vi "System_Guide-plot.vi"(6 "Time In":i32, 8 "Temperature Sync":i32, 9 "Temp Band % (e.g. 1%=1.01)":dbl=1.04, 10 "Mean(Off)/Interval(On)":bool, 11 "TempGuide":bool) -> (0 "Graph 4":dbl, 1 "Graph 3":dbl, 2 "Graph 2":dbl, 3 "Graph 1":dbl, 4 "Time out":i32)   [LabVIEW 2014]
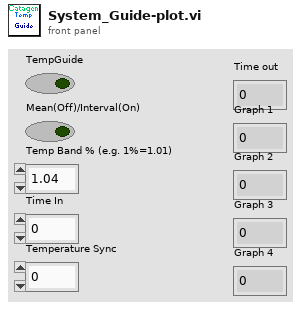
[diagram p1: front panel]
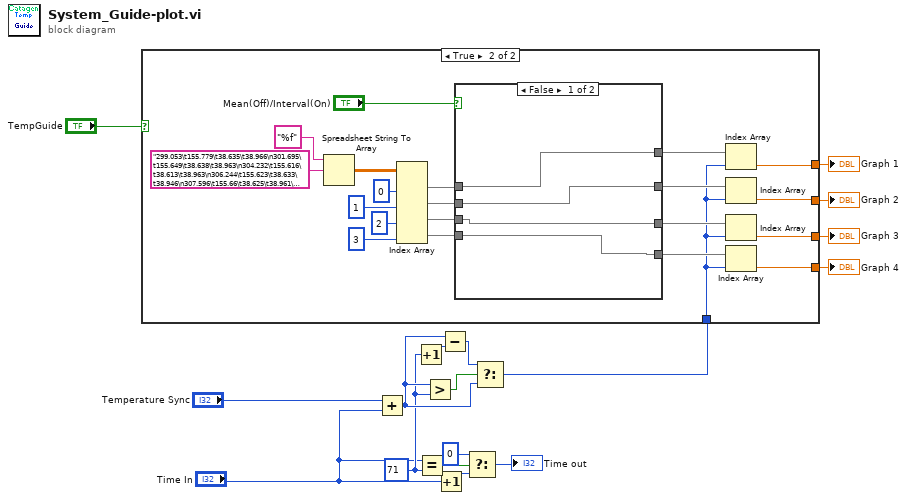
[diagram p0: block diagram]
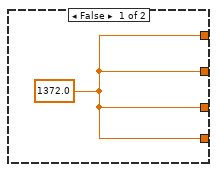
[diagram p2: hidden frame]
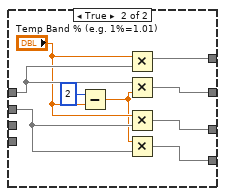
[diagram p3: hidden frame]
diagram:
  w8 = 71 ("y")
  n1 = Add(x="Temperature Sync", y="Time In") -> (x+y=w10:i32)
  n2 = Increment(x=w8) -> (x+1=w9:i32)
  n3 = Equal?(x="Time In", y=w8) -> (x = y?=w15:bool)
  n4 = Greater?(x=w10, y=w8) -> (0:w12:bool)
  n5 = Increment(x="Time In") -> (x+1=w13:i32)
  n6 = Subtract(x=w10, y=w9) -> (x-y=w11:i32)
  n7 = Select(t=0, s=w15, f=w13) -> (s? t:f=→"Time out":i32)
  n8 = Select(t=w11, s=w12, f=w10) -> (s? t:f=w7:i32)
  n9 = case shown="True" "TempGuide" {
    tunnel: w7 -> [_ w28]
    tunnel: [w18 w24] -> w4
    tunnel: [w18 w25] -> w3
    tunnel: [w18 w27] -> w2
    tunnel: [w18 w26] -> w1
    frame False {
      w18 = 1372.0
    }
    frame True {
      n10 = Spreadsheet String To Array(format string="%f", spreadsheet string="299.053\t155.779\t38.635\t38.966\n301.695\t155.649\t38.638\t38.963\n304.232\t155.616\t38.613\t38.963\n306.244\t155.623\t38.633\t38.946\n307.596\t155.66\t38.625\t38.961\n308.294\t155.857\t38.658\t38.928\n309.648\t155.893\t38.653\t38.934\n310.139\t156.057\t38.631\t38.949\n310.91\t156.073\t38.635\t38.976\n311.337\t156.182\t38.656\t38.934\n311.557\t156.297\t38.638\t38.927\n311.735\t156.496\t38.648\t38.94\n311.331\t156.331\t38.645\t38.933\n312.349\t156.573\t38.634\t38.926\n311.548\t156.657\t38.596\t38.866\n312.25\t156.94\t38.626\t38.938\n311.486\t157.037\t38.596\t38.93\n312.27\t157.108\t38.598\t38.918\n312.09\t157.285\t38.606\t38.939\n312.391\t157.179\t38.581\t38.912\n312.189\t157.496\t38.586\t38.923\n312.296\t157.418\t38.631\t38.956\n312.639\t157.483\t38.634\t38.91\n312.707\t157.778\t38.617\t38.926\n312.797\t157.869\t38.605\t38.919\n312.125\t157.953\t38.624\t38.884\n313.128\t158.062\t38.639\t38.911\n312.284\t158.157\t38.638\t38.893\n309.138\t158.378\t38.647\t38.906\n306.75\t158.387\t38.63\t38.911\n304.544\t158.237\t38.642\t38.928\n302.831\t158.006\t38.611\t38.891\n299.558\t157.813\t38.645\t38.947\n295.464\t157.413\t38.641\t38.929\n292.116\t157.055\t38.62\t38.906\n295.531\t156.58\t38.628\t38.923\n299.517\t156.284\t38.607\t38.929\n302.577\t156.271\t38.601\t38.931\n304.642\t156.227\t38.626\t38.915\n306.593\t156.238\t38.633\t38.915\n307.747\t156.343\t38.65\t38.916\n309.226\t156.368\t38.641\t38.948\n309.948\t156.588\t38.635\t38.919\n310.419\t156.708\t38.634\t38.967\n311.032\t156.802\t38.648\t39.004\n311.277\t156.957\t38.642\t38.968\n311.732\t156.994\t38.652\t38.916\n311.925\t157.11\t38.632\t38.973\n312.166\t157.279\t38.622\t38.956\n312.254\t157.296\t38.632\t38.966\n312.16\t157.492\t38.627\t38.961\n312.506\t157.536\t38.651\t38.976\n311.985\t157.508\t38.678\t38.968\n312.57\t157.727\t38.645\t38.98\n311.954\t157.632\t38.616\t38.957\n312.228\t157.895\t38.662\t38.966\n312.292\t157.836\t38.639\t38.965\n312.511\t157.872\t38.64\t38.993\n312.269\t157.969\t38.658\t38.981\n312.346\t158.137\t38.626\t38.935\n312.643\t158.208\t38.656\t38.966\n312.486\t158.2\t38.651\t38.971\n312.174\t158.203\t38.627\t38.906\n310.471\t158.505\t38.611\t38.983\n307.38\t158.432\t38.596\t38.972\n305.591\t158.343\t38.599\t38.974\n302.907\t158.133\t38.597\t38.927\n300.261\t157.782\t38.638\t38.94\n296.384\t157.418\t38.615\t38.979\n292.863\t156.943\t38.643\t38.943\n289.549\t156.606\t38.622\t39.006\n293.546\t156.064\t38.646\t39.006") -> (array=w38:dbl[][])  [unwired: 2 in]
      n11 = Index Array(array=w38, index (col) #1=0 ("disabled index (col)"), index (col) #2=1 ("disabled index (col)"), index (col) #3=2 ("index (col)"), index (col) #4=3 ("index (col)")) -> (element #1=w35:dbl[], element #2=w34:dbl[], element #3=w22:dbl[], element #4=w21:dbl[])  [unwired: 4 in]
      n12 = case shown="False" "Mean(Off)/Interval(On)" {
        tunnel: w35 -> [w43 w49]
        tunnel: w34 -> [w42 w46]
        tunnel: [w41 w44] -> w33
        tunnel: [w40 w48] -> w32
        tunnel: [w42 w50] -> w30
        tunnel: [w43 w51] -> w29
        tunnel: w22 -> [w41 _]
        tunnel: w21 -> [w40 _]
        frame False {
        }
        frame True {
          n13 = Subtract(x=2, y="Temp Band % (e.g. 1%=1.01)") -> (x-y=w45:dbl)
          n14 = Multiply(x="Temp Band % (e.g. 1%=1.01)", y=w49) -> (x*y=w51:dbl[])
          n15 = Multiply(x=w49, y=w45) -> (x*y=w50:dbl[])
          n16 = Multiply(x="Temp Band % (e.g. 1%=1.01)", y=w46) -> (x*y=w44:dbl[])
          n17 = Multiply(x=w45, y=w46) -> (x*y=w48:dbl[])
        }
      }
      n18 = Index Array(array=w29, index=w28) -> (element=w24:dbl)
      n19 = Index Array(array=w30, index=w28) -> (element=w25:dbl)
      n20 = Index Array(array=w33, index=w28) -> (element=w27:dbl)
      n21 = Index Array(array=w32, index=w28) -> (element=w26:dbl)
    }
  }
  "Graph 1" <- w4
  "Graph 2" <- w3
  "Graph 3" <- w2
  "Graph 4" <- w1
